vi "SR Status Sort.vi"(11 "list in":T1[](array[typedef]) {"Creation Date" format="%<%x>T"; "Last Updated" format="%<%x>T"}) -> (3 "Array":T1[](array[typedef]) {"Creation Date" format="%<%x>T"; "Last Updated" format="%<%x>T"})   [LabVIEW 2018]
uses:
  Type Defs/SR Cluster.ctl
  Type Defs/SR Status.ctl
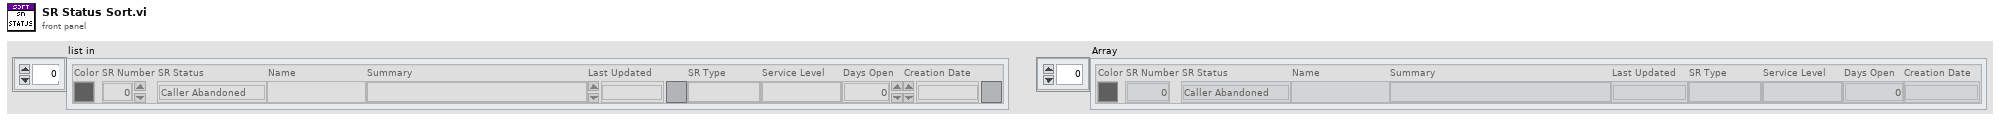
[diagram p1: front panel]
types:
  T1 = typedef "SR Cluster.ctl" = cluster{"Color":u32, "SR Number":i32, "SR Status":T2, "Name":string, "Summary":string, "Last Updated":timestamp, "SR Type":string, "Service Level":string, "Days Open":dbl, "Creation Date":timestamp}
  T2 = typedef "SR Status.ctl" = enum16{"Caller Abandoned", "Created in Error", "Expired", "Forum Resolved AE", "Forum Resolved Customer", "IN WORK", "IN WORK Collab with AES", "IN WORK Collab with PSE", "IN WORK Collab with SE", "IN WORK Customer Added Note", "IN WORK Escalation", "IN WORK Wait on Customer", "Open", "Potentially Resolved", "Presumed Resolved", "RMA Approved for Return", "RMA Closed", "RMA Closed - DOA", "RMA In Progress", "RMA Open", "RMA Waiting on Customer", "Resolved", "Passed Off"}
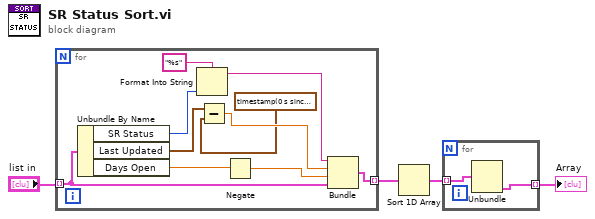
[diagram p0: block diagram]
diagram:
  n1 = for {
    tunnel: "list in" -> [w9] mode=indexing
    tunnel: [w14] -> w1 mode=indexing
    n2 = Unbundle By Name(w9) -> ("SR Status"=w13:T2, "Last Updated"=w5:timestamp, "Days Open"=w8:dbl)
    n3 = Format Into String(format string="%s", w13) -> (resulting string=w11:string)  [unwired: 2 in, 1 out]
    n4 = Subtract(x=w5, y=timestamp(0 s since 1904-01-01)) -> (x-y=w10:dbl)
    n5 = Negate(x=w8) -> (-x=w7:dbl)
    n6 = Bundle(w11, w10, w7, "SR Cluster"=w9) -> (w14:cluster{string, dbl, dbl, "SR Cluster":T1})  [unwired: 1 in]
  }
  n7 = Sort 1D Array(array=w1) -> (sorted array=w2:cluster{string, dbl, dbl, "SR Cluster":T1}[])
  n8 = for {
    tunnel: w2 -> [w16] mode=indexing
    tunnel: [w15] -> w4 mode=indexing
    n9 = Unbundle(w16) -> ("SR Cluster"=w15:T1)  [unwired: 3 out]
  }
  "Array" <- w4
